vi "ImageScan.vi"() -> ()   [LabVIEW 2017]
uses:
  ImageDisplayPropertiesDataTypeNDisplay.ctl
  ColorMapEnum.ctl
  Expose/Labview/Parameters/ExposeParameterBindingType.ctl
  617a20d7-fd07-4949-a71f-7dedcaf49b7a.vi
  ac26c0c3-9227-48f3-92c1-3e8259edfa64.vi
  3d3e9046-7624-4ffc-a947-04eb9a8f18cf.vi
  a3eee689-631a-412f-bbfa-240465c34a85.vi
  b902e6a1-dd25-4a6d-bb08-00b0fb40beac.vi
  dd66a38b-177c-4319-8bdc-72efa55adf23.vi
  6be8719f-754a-4597-a840-92194c051a39.vi
  Experiment/ExpGet.vi
  Expose/Labview/Core/ExposeInvokeMethod.vi
  <userlib>/_OpenG.lib/lvdata/lvdata.llb/Get Default Data from Variant__ogtk.vi
  88b729ff-5f39-4a55-98ec-e0f7b959dead.vi
panel:
  in  "Tab Control":enum32{"Control", "Config", "Develop"}(tab)
  in  "btnMaxRange":bool
  in  "PositionTracking":bool
  in  "positionGO":bool
  in  "Position":cluster{"X":dbl, "Y":dbl} caption="Postion" {"Y" step=0.01; "X" step=0.01}
  in  "ScanParameters":T1={"X"=0.0, "Y"=0.0, "Width"=200.0, "Height"=200.0, "Time"=3000.0, "AsDwellTime"=FALSE, "N"=500.0, "FromCenter"=TRUE, "MultiDir"=TRUE} caption="Scan" {"N" min=0.0 max=2500.0; "Time" min=0.0; "Height" min=0.0; "Width" min=0.0}
  in  "btnScan":bool
  in  "btnRegionToScan":bool
  in  "Key Step":dbl=0.2
  in  "SystemConfig":T2 caption="General System Config"
  in  "PositionConfig":T3={"UnitsToVolts"=0.02130752, "XToYRatio"=0.642, "InvertXY"=FALSE} caption="Positioner Config" {"XToYRatio" min=0.0; "UnitsToVolts" min=0.0 max=1.0}
  in  "ScanConfig":T4={"AutoAdjustRates"=TRUE, "ClockRate"=500000.0, "MeasureBinN"=20.0, "MeasureBinMinT"=200.0, "ShowStream"=TRUE, "MaxClockRate"=500000.0, "MeasureBinMaxT"=10000.0, "ScanMaxRange"=500.0, "SaveTempFiles"=TRUE, "MaxNumberOfTempFiles"=500.0} caption="Scan Device Config"
  in  "StreamConfig":T5={"ClockRate"=4000.0, "UpdateTime"=50.0, "IntegrationTime"=1.0, "CollectionWindow"=5000.0, "PadWithZeros"=FALSE, "AutoAdjustRates"=TRUE} caption="Stream Device Config" {"UpdateTime" min=5.0 max=3000.0 step=1.0}
  in  "Do Labview expose logging":bool
  in  "Disable internal matlab env.":bool=TRUE
  in  "Do Expose Logging":bool
  out "Number of bounds controls":dbl
  out "Event Hartbeat":bool
  out "Log":string
  in  "IsRFChanOpen":bool
  in  "IsLaserChanOpen":bool
  in  "btnAbort":bool
  in  "IsStreamingReader":bool
  out "ScanProgress":u8(slide) scale=0.0..100.0
  out "ReaderAmplitude":dbl format="%_7g"
  out "ExpID":string="Exp967f258c607eed45caf40f4c3101458dC" caption="Exp. ID (Debug)"
  in  "StatusFlags":T6
  out "HasBeenInitialized":bool=TRUE
  out "IsWorking":bool
  in  "FileInfo":T7
  in  "lstLastImages":u16(ring)
  in  "Colormap":T8
  in  "StreamTrace":u16[](array[numeric])
  in  "ScanImage":u16[][](array[numeric])
  out "ImageProperties":T9={"X"=0.0, "Y"=0.0, "Width"=200.0, "Height"=200.0, "FromCenter"=TRUE, "Xn"=200.0, "Yn"=200.0, "min"=0.0, "max"=200.0, "med"=200.0} caption="Current Image properties"
  in  "LoadImg":bool
  in  "btnSave":bool
  in  "IntensityLogScale":bool
  out "ImageGraph":u16[][](graph) caption="Image"
  in  "IsSavingStreamToFile":bool
  in  "StreamLogScale":bool
  out "StreamGraph":u16[](graph) caption="Stream"
  # "Display"
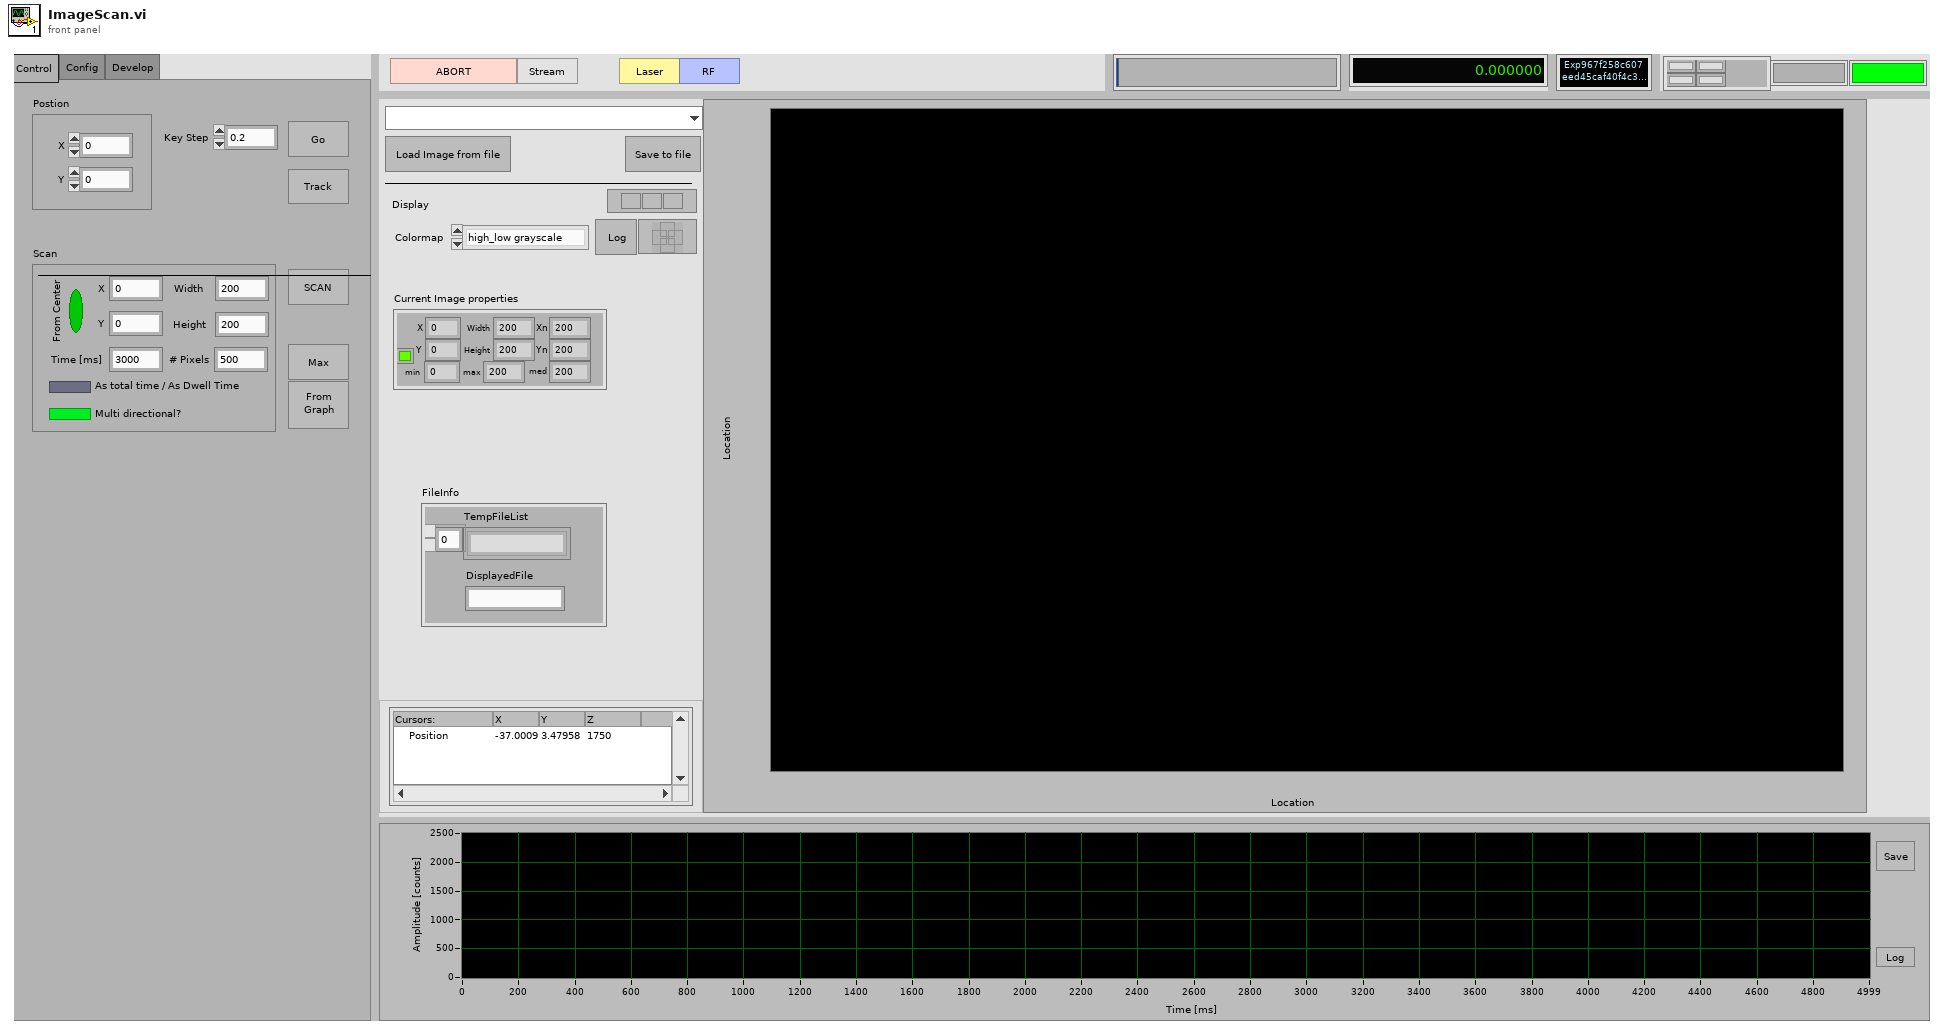
[diagram p1: front panel]
types:
  T1 = cluster{"X":dbl, "Y":dbl, "Width":dbl, "Height":dbl, "Time":dbl, "AsDwellTime":bool, "N":dbl, "FromCenter":bool, "MultiDir":bool}
  T2 = cluster{"UseAnalogInputA0":bool, "UseInternalClock":bool}
  T3 = cluster{"UnitsToVolts":dbl, "XToYRatio":dbl, "InvertXY":bool}
  T4 = cluster{"AutoAdjustRates":bool, "ClockRate":dbl, "MeasureBinN":dbl, "MeasureBinMinT":dbl, "ShowStream":bool, "MaxClockRate":dbl, "MeasureBinMaxT":dbl, "ScanMaxRange":dbl, "SaveTempFiles":bool, "MaxNumberOfTempFiles":dbl}
  T5 = cluster{"ClockRate":dbl, "UpdateTime":dbl, "IntegrationTime":dbl, "CollectionWindow":dbl, "PadWithZeros":bool, "AutoAdjustRates":bool}
  T6 = cluster{"IsStreaming":bool, "IsScanning":bool, "PossibleLossOfData":bool, "IsSettingPosition":bool}
  T7 = cluster{"TempFileList":string[], "DisplayedFile":string}
  T8 = typedef "ColorMapEnum.ctl" = enum16{"high_low grayscale", "grayscale", "jet", "high_low_winter", "None "}
  T9 = typedef "ImageDisplayPropertiesDataTypeNDisplay.ctl" = cluster{"X":dbl, "Y":dbl, "Width":dbl, "Height":dbl, "FromCenter":bool, "Xn":dbl, "Yn":dbl, "min":dbl, "max":dbl, "med":dbl}
  T10 = enum8{"Enabled", "Disabled", "Disabled and Grayed Out"}
  T11 = typedef "ExposeParameterBindingType.ctl" = enum16{"ToRemote", "FromRemote", "Bidrectional"}
  T12 = typedef "ExposeEventStreamDataType.ctl" = refnum<user-event>
  T13 = typedef "LVPoint32TypeDef.ctl" = cluster{"Horizontal":i32, "Vertical":i32}
  T14 = typedef "LVRectTypeDef.ctl" = cluster{"Left":i16, "Top":i16, "Right":i16, "Bottom":i16}
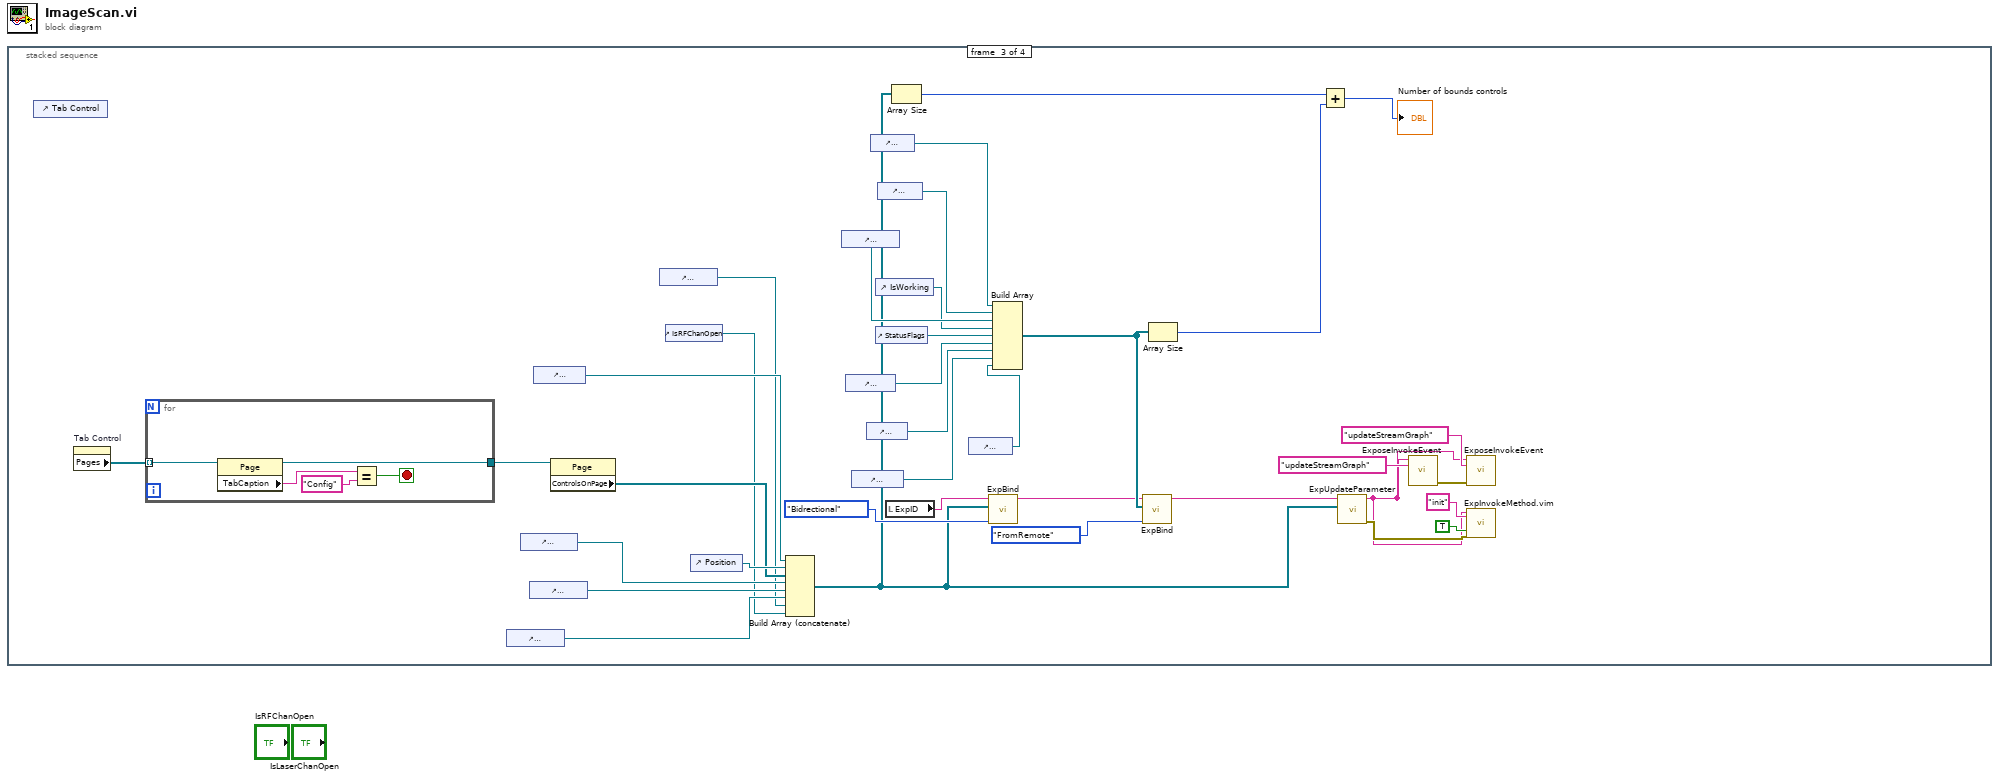
[diagram p0: block diagram]
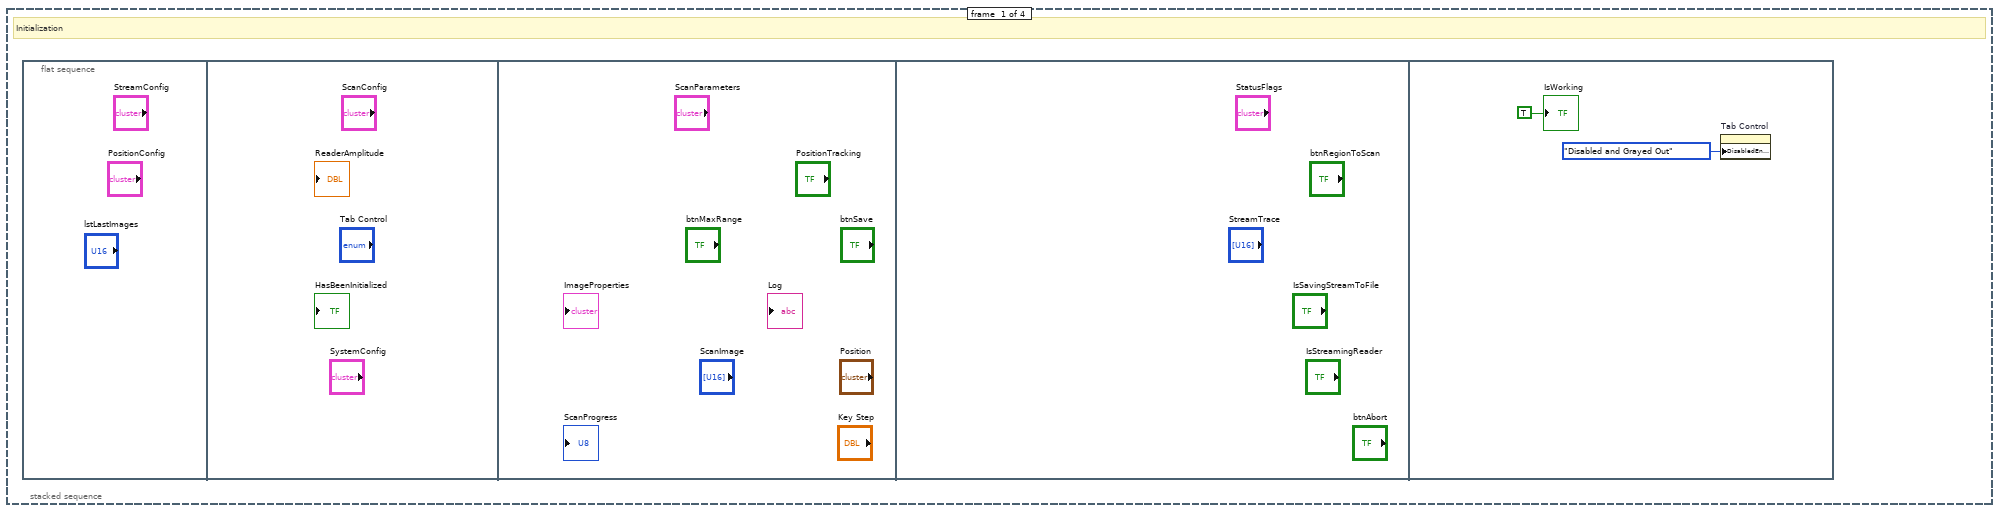
[diagram p2: hidden frame]
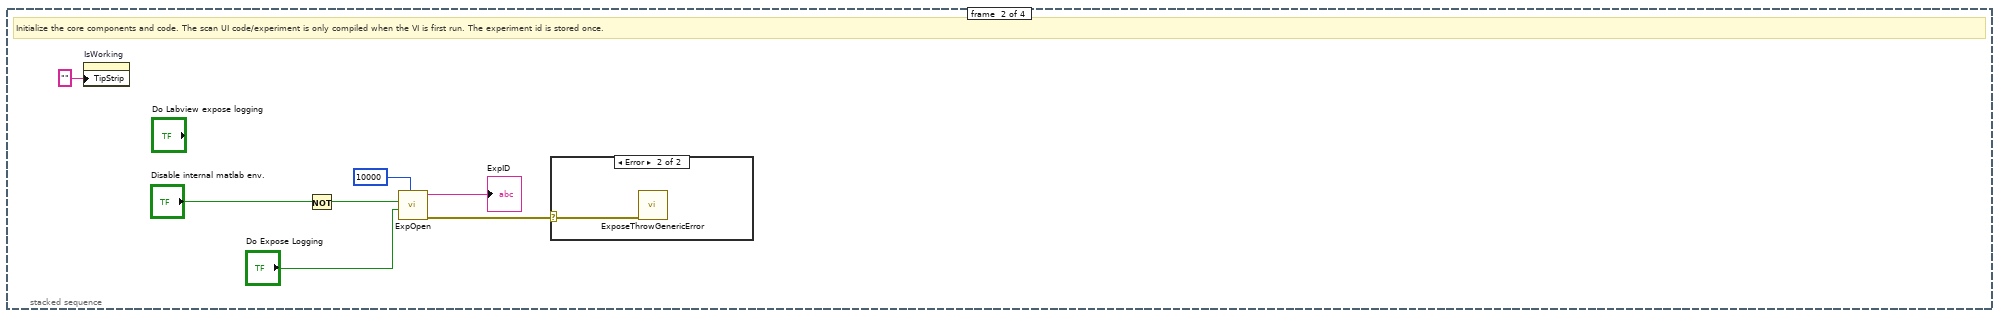
[diagram p3: hidden frame]
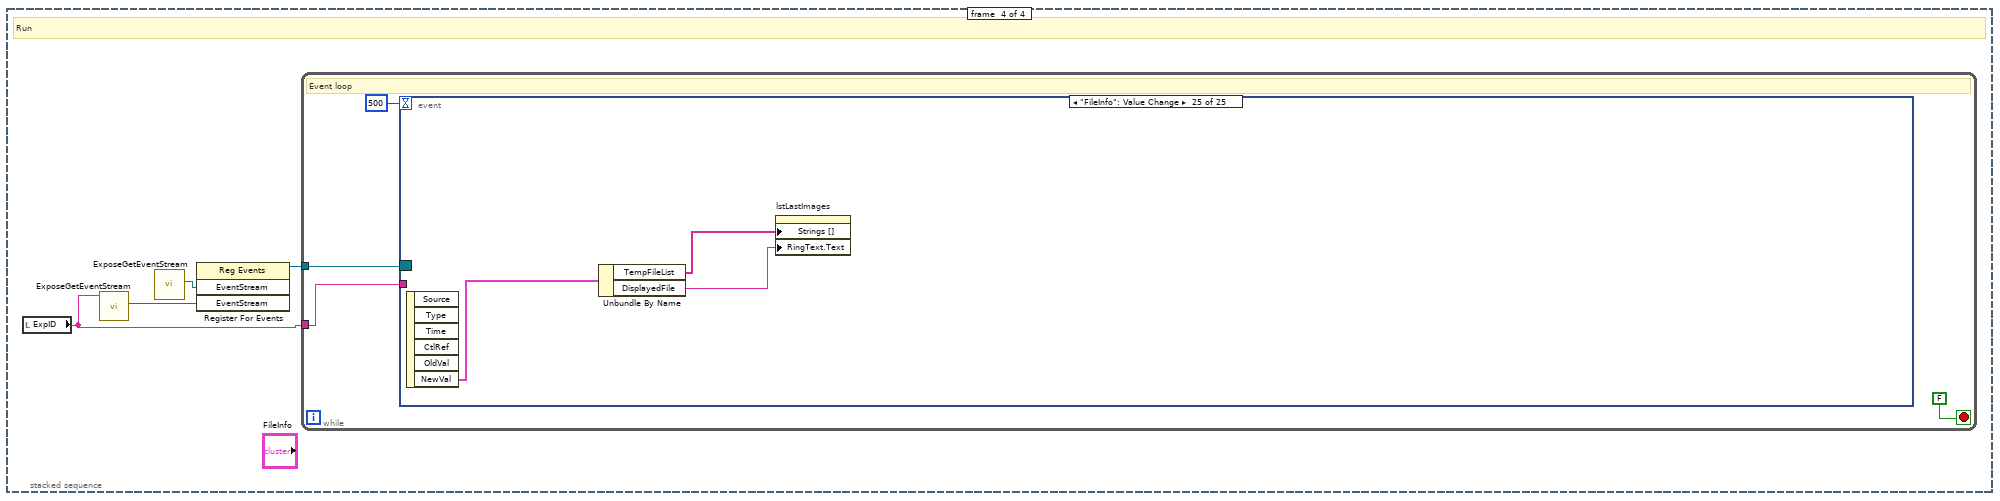
[diagram p5: hidden frame]
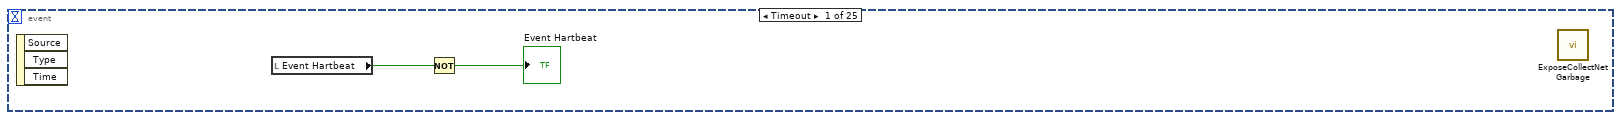
[diagram p6: hidden frame]
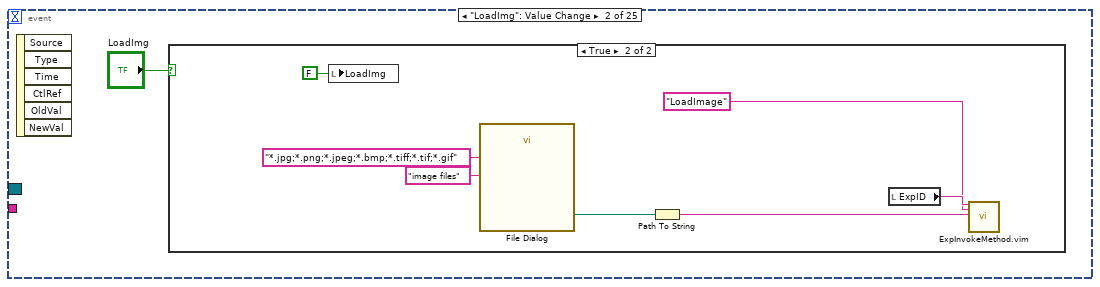
[diagram p7: hidden frame]
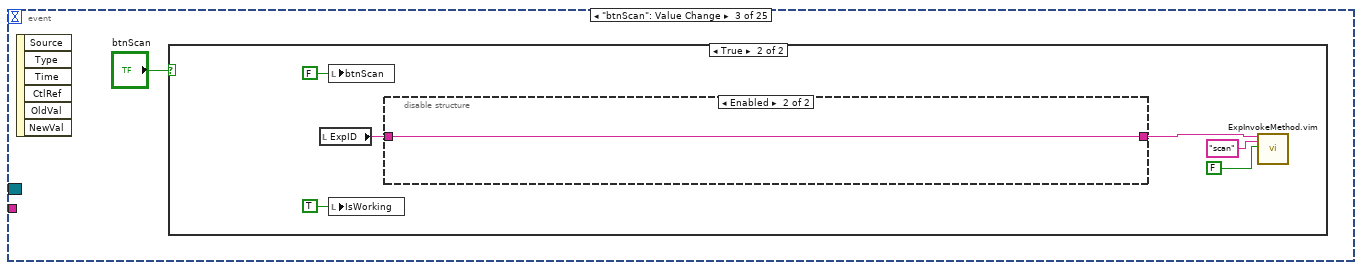
[diagram p9: hidden frame]
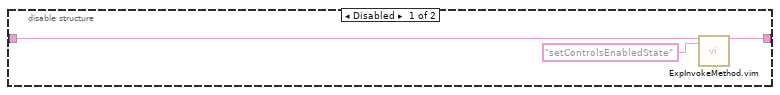
[diagram p11: hidden frame]
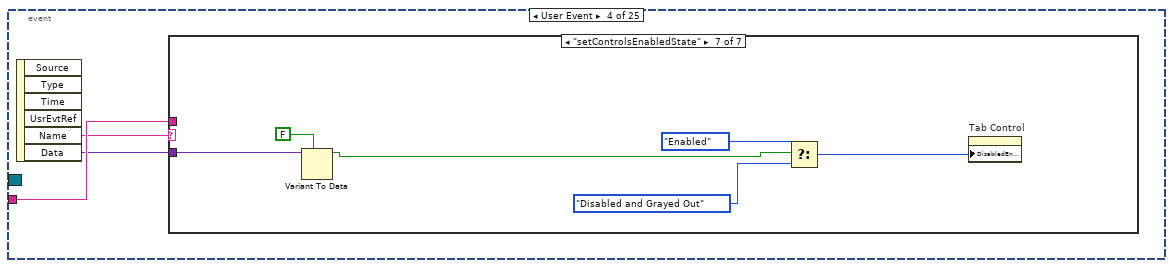
[diagram p12: hidden frame]
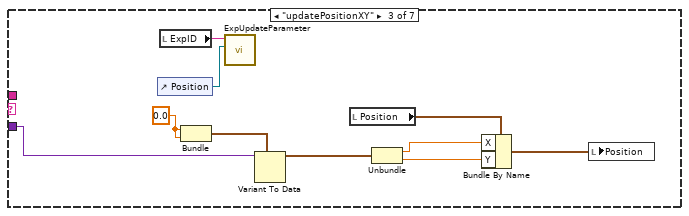
[diagram p15: hidden frame]
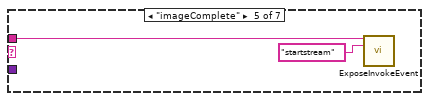
[diagram p17: hidden frame]
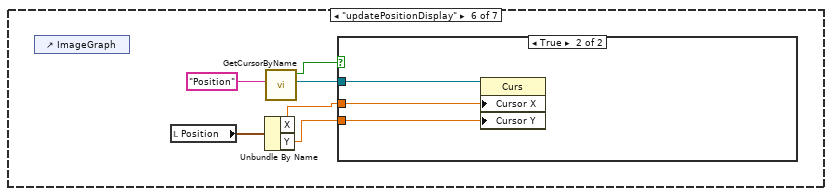
[diagram p18: hidden frame]
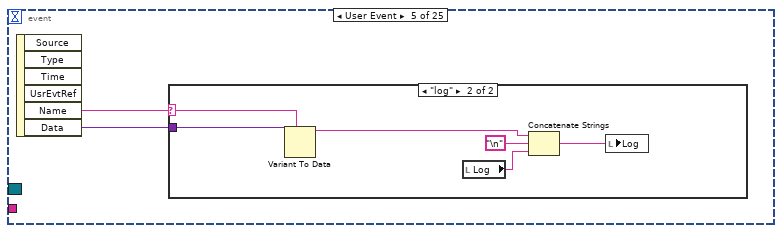
[diagram p20: hidden frame]
diagram:
  n1 = stacked-sequence {
    frame #0 {
      # "Initialization"
      n2 = flat-sequence {
        frame #0 {
        }
        frame #1 {
        }
        frame #2 {
        }
        frame #3 {
        }
        frame #4 {
          n3 = property on="Tab Control" class="TabCtl (strict)"("DisabledEnum"=T10."Disabled and Grayed Out" ("Disabled")) -> ()  [unwired: 2 in, 2 out]
          "IsWorking" <- TRUE ("Status")
        }
      }
    }
    frame #1 {
      # "Initialize the core components and code. The scan UI code/experiment is only compiled when the VI is first run. The experiment id is stored once."
      n4 = property on="IsWorking" class="Bool (strict)"("TipStrip"="" ("Tip Strip")) -> ()  [unwired: 2 in, 2 out]
      n5 = Not(x="Disable internal matlab env.") -> (.not. x?=w3:bool)
      n6 = call "ExpOpen.vi"("Timeout (ms)"=10000, "Do Expose Logging"="Do Expose Logging", "Requires Matlab Enviroment"=w3) -> ("error out"=w8:errorcluster, "ExpID"=→"ExpID":string)  [unwired: 6 in, 1 out]
      n7 = case shown="Error" w8 {
        selector: w8 -> [_ w10]
        frame No Error {
        }
        frame Error {
          n8 = call "ExposeThrowGenericError.vi"("error in (no error)"=w10) -> ()  [unwired: 10 in, 1 out]
        }
      }
    }
    frame #2 {
      n9 = control-ref of="Tab Control"() -> ()  [unwired: 1 out]
      n10 = property on="Tab Control" class="TabCtl (strict)"() -> ("Pages"=w31:refnum<vi>[])  [unwired: 2 in, 2 out]
      n11 = for {
        tunnel: w31 -> [w51] mode=indexing
        tunnel: [w47] -> w30
        stop <- w48 stop-if-true
        n12 = property class="Page"(reference=w51) -> (reference out=w47:refnum<vi>, "TabCaption"=w50:string)  [unwired: 1 in, 1 out]
        n13 = Equal?(x=w50, y="Config") -> (x = y?=w48:bool)
      }
      n14 = control-ref of="IsSavingStreamToFile"() -> (w19:refnum<vi>)
      n15 = control-ref of="IsStreamingReader"() -> (w44:refnum<vi>)
      n16 = control-ref of="PositionTracking"() -> (w39:refnum<vi>)
      n17 = control-ref of="ScanParameters"() -> (w46:refnum<vi>)
      n18 = property class="Page"(reference=w30) -> ("ControlsOnPage"=w29:refnum<vi>[])  [unwired: 1 in, 2 out]
      n19 = control-ref of="IsLaserChanOpen"() -> (w12:refnum<vi>)
      n20 = control-ref of="IsRFChanOpen"() -> (w11:refnum<vi>)
      n21 = control-ref of="Position"() -> (w45:refnum<vi>)
      n22 = Build Array (concatenate)(w46, w45, w29, w44, w39, w19, w12, w11) -> (w24:refnum<vi>[])
      n23 = control-ref of="HasBeenInitialized"() -> (w43:refnum<vi>)
      n24 = control-ref of="ReaderAmplitude"() -> (w41:refnum<vi>)
      n25 = control-ref of="ImageProperties"() -> (w22:refnum<vi>)
      n26 = control-ref of="ScanProgress"() -> (w35:refnum<vi>)
      n27 = control-ref of="StreamTrace"() -> (w20:refnum<vi>)
      n28 = control-ref of="IsWorking"() -> (w42:refnum<vi>)
      n29 = control-ref of="StatusFlags"() -> (w40:refnum<vi>)
      n30 = control-ref of="ScanImage"() -> (w21:refnum<vi>)
      n31 = local read "ExpID"() -> (w25:string)
      n32 = Array Size(array=w24) -> (size(s)=w37:i32)
      n33 = control-ref of="TempFileList"() -> (w13:refnum<vi>)
      n34 = call "ExpBind.vi"("Binding Type"=ExposeParameterBindingType."Bidrectional", "Value"=w24, "ExpID"=w25) -> ("ExpID out"=w16:string)  [unwired: 7 in, 1 out]
      n35 = Build Array(w20, w21, w43, w42, w40, w41, w35, w22, w13) -> (w27:refnum<vi>[])
      n36 = call "ExpBind.vi"("Binding Type"=ExposeParameterBindingType."FromRemote", "Value"=w27, "ExpID"=w16) -> ("ExpID out"=w15:string)  [unwired: 7 in, 1 out]
      n37 = Array Size(array=w27) -> (size(s)=w38:i32)
      n38 = Add(x=w37, y=w38) -> (x+y=→"Number of bounds controls":i32)
      n39 = call "ExpUpdateParameter.vi"("Variant"=w24, "ExpID"=w15) -> ("error out"=w17:errorcluster, "ExpID out"=w14:string)  [unwired: 8 in]
      n40 = call "ExposeInvokeEvent.vi"("ID"=w14, "name"="updateStreamGraph" ("eventName")) -> ("error out"=w18:errorcluster)  [unwired: 13 in]
      n41 = call "ExposeInvokeEvent.vi"("ID"=w14, "name"="updateStreamGraph" ("eventName"), "error in (no error)"=w18) -> ()  [unwired: 12 in, 1 out]
      n42 = call "ExpInvokeMethod.vim"("ExpID"=w14, "Method Name"="init" ("event data"), "Require Response"=TRUE, "error in (no error)"=w17) -> ()  [unwired: 13 in, 3 out]
    }
    frame #3 {
      # "Run"
      n43 = local read "ExpID"() -> (w55:string)
      n44 = call "ExposeGetEventStream.vi"("ID"=w55) -> ("EventStream"=w53:T12)  [unwired: 7 in, 3 out]
      n45 = call "ExposeGetEventStream.vi"() -> ("EventStream"=w54:T12)  [unwired: 8 in, 3 out]
      n46 = register-events(w54, w53) -> (reference out=w52:refnum<event-registration>)  [unwired: 2 in, 1 out]
      n47 = while {
        tunnel: w55 -> [w57]
        tunnel: w52 -> [w56]
        stop <- FALSE stop-if-true
        # "Event loop"
        n48 = event shown="[24] \"FileInfo\": Value Change" {
          selector: w56 -> [_ _ _ _ _ _ _ _ _ _ _ _ _ _ _ _ _ _ _ _ _ _ _ _ _]
          dyn-events: _ -> [_ _ _ _ _ _ _ _ _ _ _ _ _ _ _ _ _ _ _ _ _ _ _ _ _]
          timeout: 500 -> [_ _ _ _ _ _ _ _ _ _ _ _ _ _ _ _ _ _ _ _ _ _ _ _ _]
          tunnel: w57 -> [_ _ _ w83 _ _ _ _ _ _ _ w169 _ _ _ w218 _ _ _ _ _ _ _ w258 _]
          event Timeout {
            n49 = event-data() -> ()  [unwired: 1 in, 3 out]
            n50 = local read "Event Hartbeat"() -> (w60:bool)
            n51 = Not(x=w60) -> (.not. x?=→"Event Hartbeat":bool)
            n52 = call "ExposeCollectNetGarbage.vi"() -> ()  [unwired: 11 in, 1 out]
          }
          event "LoadImg": Value Change {
            n53 = event-data() -> ()  [unwired: 1 in, 6 out]
            n54 = case shown="True" "LoadImg" {
              frame False {
              }
              frame True {
                n55 = local write "LoadImg"(FALSE ("LoadImg")) -> ()
                n56 = call "File Dialog"("pattern (all files)"="*.jpg;*.png;*.jpeg;*.bmp;*.tiff;*.tif;*.gif", "pattern label"="image files") -> ("selected path"=w68:path)  [unwired: 10 in, 3 out]
                n57 = Path To String(path=w68) -> (string=w67:string)
                n58 = local read "ExpID"() -> (w66:string)
                n59 = call "ExpInvokeMethod.vim"("ExpID"=w66, "Method Name"="LoadImage", "Argument(s)"=w67) -> ()  [unwired: 14 in, 3 out]
              }
            }
          }
          event "btnScan": Value Change {
            n60 = event-data() -> ()  [unwired: 1 in, 6 out]
            n61 = case shown="True" "btnScan" {
              frame False {
              }
              frame True {
                n62 = local read "ExpID"() -> (w74:string)
                n63 = local write "btnScan"(FALSE ("ScanBtn")) -> ()
                n64 = local write "IsWorking"(TRUE ("IsWorking")) -> ()
                n65 = disable-structure shown="Enabled" {
                  disable-tunnel: w74 -> [w79 w80]
                  disable-tunnel: [w78 w80] -> w73
                  frame Disabled {
                    n66 = call "ExpInvokeMethod.vim"("ExpID"=w79, "Method Name"="setControlsEnabledState" ("eventName")) -> ("ExpID out"=w78:string)  [unwired: 15 in, 2 out]
                  }
                  frame Enabled {
                  }
                }
                n67 = call "ExpInvokeMethod.vim"("ExpID"=w73, "Method Name"="scan", "Argument(s)"=FALSE) -> ()  [unwired: 14 in, 3 out]
              }
            }
          }
          event User Event {
            n68 = event-data() -> ("Name"=w82:string, "Data"=w81:variant)  [unwired: 1 in, 4 out]
            n69 = case shown="\"setControlsEnabledState\"" w82 {
              tunnel: w81 -> [_ _ w91 _ _ _ w110]
              tunnel: w83 -> [_ _ _ _ w94 _ _]
              frame "False", Default {
              }
              frame "startstream" {
              }
              frame "updatePositionXY" {
                w93 = 0.0
                n70 = control-ref of="Position"() -> (w84:refnum<vi>)
                n71 = local read "ExpID"() -> (w85:string)
                n72 = Bundle(w93, w93) -> (w92:cluster{dbl, dbl})  [unwired: 1 in]
                n73 = call "ExpUpdateParameter.vi"("Variant"=w84, "ExpID"=w85) -> ()  [unwired: 8 in, 2 out]
                n74 = Variant To Data(type=w92, Variant=w91) -> (data=w90:cluster{dbl, dbl})  [unwired: 1 in, 1 out]
                n75 = local read "Position"() -> (w89:cluster{"X":dbl, "Y":dbl})
                n76 = Unbundle(w90) -> (w88:dbl, w87:dbl)
                n77 = Bundle By Name(cluster=w89, "X"=w88, "Y"=w87) -> (w86:cluster{"X":dbl, "Y":dbl})
                n78 = local write "Position"(w86) -> ()
              }
              frame "updateAvailableExperiments" {
              }
              frame "imageComplete" {
                n79 = call "ExposeInvokeEvent.vi"("ID"=w94, "name"="startstream" ("event data")) -> ()  [unwired: 13 in, 1 out]
              }
              frame "updatePositionDisplay" {
                n80 = control-ref of="ImageGraph"() -> ()  [unwired: 1 out]
                n81 = local read "Position"() -> (w96:cluster{"X":dbl, "Y":dbl})
                n82 = Unbundle By Name(w96) -> ("X"=w100:dbl, "Y"=w99:dbl)
                n83 = call "GetCursorByName.vi"("Name"="Position") -> ("CursorRef"=w98:refnum<vi>, "Found?"=w97:bool)  [unwired: 8 in, 1 out]
                n84 = case shown="True" w97 {
                  tunnel: w100 -> [_ w104]
                  tunnel: w99 -> [_ w103]
                  tunnel: w98 -> [_ w102]
                  frame False {
                  }
                  frame True {
                    n85 = property class="Curs"(reference=w102, "Cursor X"=w104, "Cursor Y"=w103) -> ()  [unwired: 1 in, 2 out]
                  }
                }
              }
              frame "setControlsEnabledState" {
                n86 = Variant To Data(type=FALSE, Variant=w110) -> (data=w108:bool)  [unwired: 1 in, 1 out]
                n87 = Select(t=T10."Enabled" ("Disabled"), s=w108, f=T10."Disabled and Grayed Out" ("Disabled")) -> (s? t:f=w105:T10)
                n88 = property on="Tab Control" class="TabCtl (strict)"("DisabledEnum"=w105) -> ()  [unwired: 2 in, 2 out]
              }
            }
          }
          event User Event {
            n89 = event-data() -> ("Name"=w112:string, "Data"=w111:variant)  [unwired: 1 in, 4 out]
            n90 = case shown="\"log\"" w112 {
              selector: w112 -> [_ w117]
              tunnel: w111 -> [_ w118]
              frame "False", Default {
              }
              frame "log" {
                n91 = Variant To Data(type=w117, Variant=w118) -> (data=w116:string)  [unwired: 1 in, 1 out]
                n92 = local read "Log"() -> (w114:string)
                n93 = Concatenate Strings(w116, "\n", w114) -> (w113:string)
                n94 = local write "Log"(w113) -> ()
              }
            }
          }
          event "ScanImage": Value Change {
            n95 = event-data() -> ("NewVal"=w119:u16[][])  [unwired: 1 in, 5 out]
            n96 = flat-sequence {
              tunnel: w119 -> [w120]
              frame #0 {
                "ImageGraph" <- w120
              }
              frame #1 {
                n97 = local read "ImageProperties"() -> (w124:T9)
                n98 = control-ref of="ImageGraph"() -> (w125:refnum<vi>)
                n99 = call "UpdateImageDisplayGraph.vi"("Graph Refnum"=w125, "ImageProperties"=w124) -> ()  [unwired: 14 in]
                n100 = Unbundle By Name(w124) -> ("min"=w123:dbl, "max"=w121:dbl, "med"=w122:dbl)
                n101 = call "ColormapToIntensityGraphZMarkers.vi"("Colormap"="Colormap", "Min"=w123, "Median"=w122, "Max"=w121) -> ("Z Scale.Marker Values[]"=w126:cluster{dbl, u32}[])  [unwired: 11 in]
                n102 = property class="IntGraph (strict)"(reference=w125, "ZScale.MarkerVals[]"=w126) -> ()  [unwired: 1 in, 2 out]
              }
            }
          }
          event Value Change {
            n103 = event-data() -> ("OldVal"=w130:T8, "NewVal"=w129:T8)  [unwired: 1 in, 4 out]
            n104 = Not Equal?(x=w130, y=w129) -> (x != y?=w128:bool)
            n105 = case shown="True" w128 {
              frame False {
              }
              frame True {
                n106 = local read "ImageProperties"() -> (w134:T9)
                n107 = Unbundle By Name(w134) -> ("min"=w133:dbl, "max"=w131:dbl, "med"=w132:dbl)
                n108 = local read "Colormap"() -> (w136:T8)
                n109 = call "ColormapToIntensityGraphZMarkers.vi"("Colormap"=w136, "Min"=w133, "Median"=w132, "Max"=w131) -> ("Z Scale.Marker Values[]"=w135:cluster{dbl, u32}[])  [unwired: 11 in]
                n110 = property on="ImageGraph" class="IntGraph (strict)"("ZScale.MarkerVals[]"=w135) -> ()  [unwired: 2 in, 2 out]
              }
            }
          }
          event "btnSave": Value Change {
            n111 = event-data() -> ("NewVal"=w138:bool)  [unwired: 1 in, 5 out]
            n112 = local write "btnSave"(FALSE ("btnSave")) -> ()
            n113 = case shown="True" w138 {
              frame False {
              }
              frame True {
                n114 = call "SelectImageToSaveTo"("pattern (all files)"="*.png") -> ("selected path"=w141:path)  [unwired: 11 in, 3 out]
                n115 = Path To String(path=w141) -> (string=w143:string)
                n116 = local read "ExpID"() -> (w139:string)
                n117 = call "ExpInvokeMethod.vim"("ExpID"=w139, "Method Name"="SaveScanToImage", "Argument(s)"=w143) -> ()  [unwired: 14 in, 3 out]
              }
            }
          }
          event "ImageGraph": Scale Range Change {
            n118 = event-data() -> ()  [unwired: 1 in, 8 out]
            n119 = control-ref of="ImageGraph"() -> (w144:refnum<vi>)
            n120 = call "AutoAdjustGraphAspectRatio.vi"("IntensityGraph in"=w144) -> ()  [unwired: 11 in]
          }
          event "btnRegionToScan": Value Change {
            n121 = event-data() -> ("NewVal"=w146:bool)  [unwired: 1 in, 5 out]
            n122 = local write "btnRegionToScan"(FALSE ("btnRegionToScan")) -> ()
            n123 = case shown="True" w146 {
              frame False {
              }
              frame True {
                n124 = control-ref of="ImageGraph"() -> (w157:refnum<vi>)
                n125 = property on="Property Node" class="IntGraph (strict)"(reference=w157) -> ("XScale.Maximum"=w156:dbl, "XScale.Minimum"=w155:dbl, "YScale.Maximum"=w154:dbl, "YScale.Minimum"=w153:dbl)  [unwired: 1 in, 2 out]
                n126 = formula code="float32 w,h,x0,y0,sqr;\nw=xmax-xmin;\nh=ymax-ymin;\nif(w>h)\n    sqr=h;\nelse\n    sqr=w;\nx0=(xmax+xmin)/2;\ny0=(ymax+ymin)/2;"("xmax"=w156, "xmin"=w155, "ymax"=w154, "ymin"=w153) -> ("sqr"=w150:sgl, "x0"=w149:sgl, "y0"=w148:sgl)
                n127 = local read "ScanParameters"() -> (w152:T1)
                n128 = Bundle By Name(cluster=w152, "X"=w149, "Y"=w148, "Width"=w150, "Height"=w150, "FromCenter"=TRUE) -> (w147:T1)
                n129 = property on="ScanParameters" class="Clust (strict)"("Val(Sgnl)"=w147) -> ()  [unwired: 2 in, 2 out]
              }
            }
          }
          event "btnMaxRange": Value Change {
            n130 = event-data() -> ("NewVal"=w159:bool)  [unwired: 1 in, 5 out]
            n131 = local write "btnMaxRange"(FALSE ("btnMaxRange")) -> ()
            n132 = case shown="True" w159 {
              frame False {
              }
              frame True {
                w161 = 0.0 ("X")
                n133 = local read "ScanParameters"() -> (w164:T1)
                n134 = property on="ScanMaxRange" class="DigNum (strict)"() -> ("Value"=w162:dbl)  [unwired: 2 in, 2 out]
                n135 = Bundle By Name(cluster=w164, "X"=w161, "Y"=w161, "Width"=w162, "Height"=w162, "FromCenter"=TRUE) -> (w160:T1)
                n136 = property on="ScanParameters" class="Clust (strict)"("Val(Sgnl)"=w160) -> ()  [unwired: 2 in, 2 out]
              }
            }
          }
          event "IsSavingStreamToFile": Value Change {
            n137 = event-data() -> ("OldVal"=w167:bool, "NewVal"=w168:bool)  [unwired: 1 in, 4 out]
            n138 = Not(x=w167) -> (.not. x?=w166:bool)
            n139 = And(x=w166, y=w168) -> (x .and. y?=w165:bool)
            n140 = case shown="True" w165 {
              tunnel: w169 -> [_ w170]
              frame False {
              }
              frame True {
                n141 = call "SelectImageToSaveTo2"("pattern (all files)"="*.mat") -> ("selected path"=w172:path)  [unwired: 11 in, 3 out]
                n142 = Path To String(path=w172) -> (string=w174:string)
                n143 = call "ExpInvokeMethod.vim"("ExpID"=w170, "Method Name"="SetStreamSaveFile", "Argument(s)"=w174) -> ()  [unwired: 14 in, 3 out]
              }
            }
          }
          event Key Down {
            n144 = event-data() -> ("ScanCode"=w181:i16)  [unwired: 1 in, 7 out]
            n145 = local read "Key Step"() -> (w180:dbl)
            n146 = case shown="72" w181 {
              tunnel: [0.0 ("Key Step") 0.0 ("Key Step") w196 w199 0.0 ("Key Step")] -> w175
              tunnel: [0.0 ("Key Step") w194 0.0 ("Key Step") 0.0 ("Key Step") w201] -> w176
              tunnel: w180 -> [_ w194 w197 w199 w202]
              frame Default {
              }
              frame 72 {
              }
              frame 75 {
                n147 = Negate(x=w197) -> (-x=w196:dbl)
              }
              frame 77 {
              }
              frame 80 {
                n148 = Negate(x=w202) -> (-x=w201:dbl)
              }
            }
            n149 = Not Equal To 0?(x=w175) -> (x != 0?=w178:bool)
            n150 = Not Equal To 0?(x=w176) -> (x != 0?=w179:bool)
            n151 = Or(x=w178, y=w179) -> (x .or. y?=w177:bool)
            n152 = case shown="True" w177 {
              tunnel: w176 -> [_ w184]
              tunnel: w175 -> [_ w182]
              frame False {
              }
              frame True {
                n153 = local read "Position"() -> (w191:cluster{"X":dbl, "Y":dbl})
                n154 = Unbundle By Name(w191) -> ("X"=w186:dbl, "Y"=w187:dbl)
                n155 = Add(x=w186, y=w182) -> (x+y=w183:dbl)
                n156 = Add(x=w187, y=w184) -> (x+y=w190:dbl)
                n157 = Bundle(w183, w190) -> (w189:cluster{dbl, dbl})  [unwired: 1 in]
                n158 = local read "ExpID"() -> (w188:string)
                n159 = call "ExposeInvokeEvent.vi"("ID"=w188, "name"="updatePositionXY", "Data"=w189) -> ()  [unwired: 12 in, 1 out]
              }
            }
          }
          event "IsWorking": Value Change {
            n160 = event-data() -> ()  [unwired: 1 in, 6 out]
            n161 = local read "IsWorking"() -> (w205:bool)
            n162 = Not(x=w205) -> (.not. x?=w204:bool)
            n163 = local read "ExpID"() -> (w207:string)
            n164 = call "ExposeInvokeEvent.vi"("ID"=w207, "name"="setControlsEnabledState" ("eventName"), "Data"=w204) -> ()  [unwired: 12 in, 1 out]
          }
          event "StreamTrace": Value Change {
            n165 = event-data() -> ("NewVal"=→"StreamGraph":u16[])  [unwired: 1 in, 5 out]
            n166 = local read "StreamConfig"() -> (w214:T5)
            n167 = Unbundle By Name(w214) -> ("IntegrationTime"=w212:dbl, "CollectionWindow"=w213:dbl, "PadWithZeros"=w210:bool)
            n168 = case shown="False" w210 {
              tunnel: w213 -> [_ w217]
              tunnel: w212 -> [_ w216]
              frame False {
              }
              frame True {
                w215 = 0.0 ("X Scale.Offset and Multiplier:Offset")
                n169 = property on="StreamGraph" class="WFGraph (strict)"("XScale.Multiplier"=w216, "XScale.Offset"=w215, "XScale.Minimum"=w215, "XScale.Maximum"=w217) -> ()  [unwired: 2 in, 2 out]
              }
            }
            n170 = Not(x=w210) -> (.not. x?=w209:bool)
            n171 = Boolean To (0,1)(Boolean=w209) -> (0, 1=w208:i16)
            n172 = property on="StreamGraph" class="WFGraph (strict)"("XScale.ScaleFit"=w208) -> ()  [unwired: 2 in, 2 out]
          }
          event "btnAbort": Value Change {
            n173 = event-data() -> ("NewVal"=w219:bool)  [unwired: 1 in, 5 out]
            n174 = case shown="True" w219 {
              tunnel: w218 -> [_ w221]
              frame False {
              }
              frame True {
                n175 = call "ExpInvokeMethod.vim"("ExpID"=w221, "Method Name"="stop") -> ()  [unwired: 15 in, 3 out]
                n176 = local write "btnAbort"(FALSE ("btnAbort")) -> ()
              }
            }
          }
          event "Position": Value Change {
            n177 = event-data() -> ()  [unwired: 1 in, 6 out]
          }
          event "ImageGraph": Mouse Up {
            n178 = event-data() -> ("Coords"=w224:T13)  [unwired: 1 in, 7 out]
            n179 = property on="ImageGraph" class="IntGraph (strict)"() -> ("Plot Bounds"=w226:T14)  [unwired: 2 in, 2 out]
            n180 = invoke on="ImageGraph" class="IntGraph (strict)" method="Map Coords To XY"("Coords"=w224) -> ("XY"=w223:cluster{"X":dbl, "Y":dbl})  [unwired: 6 in, 6 out]
            n181 = call <vilib>:"PointInRect.vi"("rect"=w226, "point"=w224) -> ("pt in rect"=w225:bool)
            n182 = case shown="True" w225 {
              tunnel: w223 -> [_ w228]
              tunnel: w223 -> [_ w227]
              frame False {
              }
              frame True {
                n183 = property on="ImageGraph" class="IntGraph (strict)"("Cursor.Cursor Position"=w228) -> ()  [unwired: 2 in, 2 out]
                n184 = property on="ImageGraph" class="IntGraph (strict)"() -> ("Cursor.Cursor Name"=w231:string)  [unwired: 2 in, 2 out]
                n185 = Equal?(x=w231, y="Position") -> (x = y?=w229:bool)
                n186 = case shown="True" w229 {
                  tunnel: w228 -> [_ _]
                  tunnel: w227 -> [_ w233]
                  frame False {
                  }
                  frame True {
                    n187 = Unbundle(w233) -> ("X"=w235:dbl, "Y"=w236:dbl)
                    n188 = local read "Position"() -> (w234:cluster{"X":dbl, "Y":dbl})
                    n189 = Bundle By Name(cluster=w234, "X"=w235, "Y"=w236) -> (w232:cluster{"X":dbl, "Y":dbl})
                    n190 = property on="Position" class="Clust (strict)"("Val(Sgnl)"=w232) -> ()  [unwired: 2 in, 2 out]
                  }
                }
              }
            }
          }
          event "StreamLogScale": Value Change {
            n191 = event-data() -> ()  [unwired: 1 in, 6 out]
            n192 = flat-sequence {
              frame #0 {
                n193 = Boolean To (0,1)(Boolean="StreamLogScale") -> (0, 1=w237:i16)
                n194 = property on="StreamGraph" class="WFGraph (strict)"("YScale.Mapping Mode"=w237) -> ()  [unwired: 2 in, 2 out]
              }
              frame #1 {
                n195 = local read "StreamGraph"() -> (w239:u16[])
                n196 = property on="StreamGraph" class="WFGraph (strict)"("Val(Sgnl)"=w239) -> ()  [unwired: 2 in, 2 out]
              }
            }
          }
          event "IntensityLogScale": Value Change {
            n197 = event-data() -> ()  [unwired: 1 in, 6 out]
            n198 = property on="ImageGraph" class="IntGraph (strict)"() -> ("Value"=w240:u16[][])  [unwired: 2 in, 2 out]
            n199 = property on="ImageGraph" class="IntGraph (strict)"("Val(Sgnl)"=w240) -> ()  [unwired: 2 in, 2 out]
            n200 = Boolean To (0,1)(Boolean="IntensityLogScale") -> (0, 1=w241:i16)
            n201 = property on="ImageGraph" class="IntGraph (strict)"("ZScale.Mapping Mode"=w241) -> ()  [unwired: 2 in, 2 out]
          }
          event "ImageGraph": Cursor Move {
            n202 = event-data() -> ("CursRef"=w247:refnum<vi>)  [unwired: 1 in, 7 out]
            n203 = property class="Curs"(reference=w247) -> (reference out=w244:refnum<vi>, "Cursor Name"=w245:string)  [unwired: 1 in, 1 out]
            n204 = Equal?(x=w245, y="Position") -> (x = y?=w243:bool)
            n205 = case shown="True" w243 {
              tunnel: w244 -> [_ w252]
              frame False {
              }
              frame True {
                n206 = property class="Curs"(reference=w252) -> ("Cursor X"=w250:dbl, "Cursor Y"=w249:dbl)  [unwired: 1 in, 2 out]
                n207 = local read "Position"() -> (w251:cluster{"X":dbl, "Y":dbl})
                n208 = Bundle By Name(cluster=w251, "X"=w250, "Y"=w249) -> (w248:cluster{"X":dbl, "Y":dbl})
                n209 = property on="Position" class="Clust (strict)"("Val(Sgnl)"=w248) -> ()  [unwired: 2 in, 2 out]
              }
            }
          }
          event "positionGO": Value Change {
            n210 = event-data() -> ()  [unwired: 1 in, 6 out]
            n211 = case shown="True" "positionGO" {
              frame False {
              }
              frame True {
                n212 = local write "positionGO"(FALSE ("positionGO")) -> ()
                n213 = local read "ExpID"() -> (w255:string)
                n214 = call "ExpInvokeMethod.vim"("ExpID"=w255, "Method Name"="sendPositionToDevice" ("event data")) -> ()  [unwired: 15 in, 3 out]
              }
            }
          }
          event Panel Close {
            n215 = event-data() -> ()  [unwired: 1 in, 4 out]
            n216 = Stop(stop? (T)=TRUE) -> ()
          }
          event "StreamConfig": Value Change {
            n217 = event-data() -> ()  [unwired: 1 in, 6 out]
            n218 = call "ExposeInvokeEvent.vi"("ID"=w258, "name"="updateStreamGraph" ("eventName")) -> ()  [unwired: 13 in, 1 out]
          }
          event "FileInfo": Value Change {
            n219 = event-data() -> ("NewVal"=w262:T7)  [unwired: 1 in, 5 out]
            n220 = Unbundle By Name(w262) -> ("TempFileList"=w261:string[], "DisplayedFile"=w260:string)
            n221 = property on="lstLastImages" class="Ring (strict)"("Strings []"=w261, "RingText.Text"=w260) -> ()  [unwired: 2 in, 2 out]
          }
        }
      }
    }
  }
